vi "Build_Asylum_Stop.vi"(8 "error in (no error)":errorcluster) -> (0 "error out":errorcluster, 3 "Command":string)   [LabVIEW 2020]
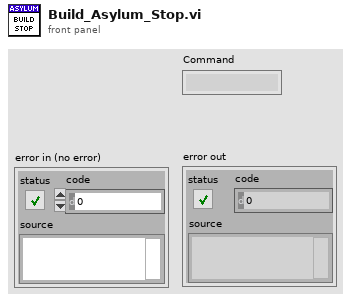
[diagram p1: front panel]
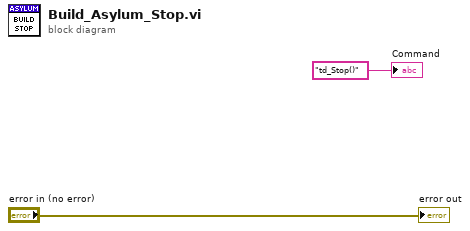
[diagram p0: block diagram]
diagram:
  "error out" <- "error in (no error)"
  "Command" <- "td_Stop()"
